vi "Test DISCONNECT packet.vi"(8 "error in":errorcluster) -> (0 "error out":errorcluster)   [LabVIEW 2013]
uses:
  source/Control Packets/DISCONNECT/DISCONNECT.lvclass
  source/Control Packets/ControlPacket/ControlPacket.lvclass/ControlPacket.ctl
  source/Control Packets/ControlPacket/ControlPacket.lvclass
  <vilib>/addons/_JKI Toolkits/Caraya/classes/Test/Test.lvclass
  <vilib>/addons/_JKI Toolkits/Caraya/classes/Assert/Assert.lvclass
panel:
  out "Packet ID":u16 format="%04x"
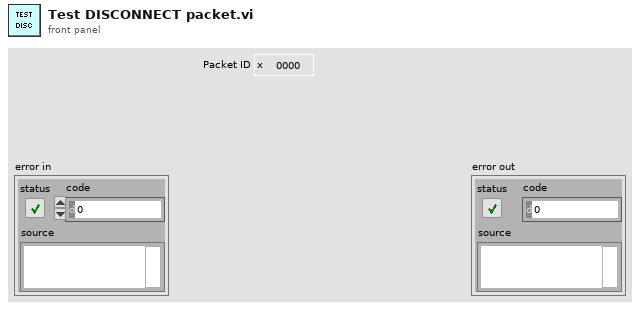
[diagram p1: front panel]
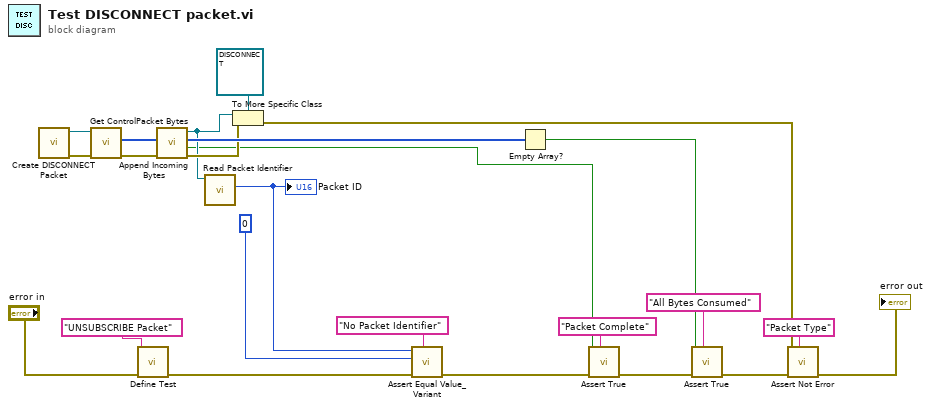
[diagram p0: block diagram]
diagram:
  n1 = call "Create DISCONNECT Packet.vi"() -> ("error out"=w18:errorcluster, "DISCONNECT"=w19:refnum<class "DISCONNECT.lvclass">)  [unwired: 10 in]
  n2 = call "Get ControlPacket Bytes.vi"("error in (no error)"=w18, "ControlPacket"=w19) -> ("error out"=w22:errorcluster, "Bytes Stream"=w24:u8[])  [unwired: 6 in, 2 out]
  n3 = call <vilib>:"Define Test.vi"("error in (no error)"="error in", "Label (VI Title)"="UNSUBSCRIBE Packet") -> ("error out"=w11:errorcluster)  [unwired: 9 in]
  n4 = call "Append Incoming Bytes.vi"("error in (no error)"=w22, "Incoming Packets"=w24) -> ("error out"=w21:errorcluster, "Complete Packet"=w4:bool, "Remaining Packets"=w23:u8[], "ControlPacket"=w20:refnum<class "ControlPacket.lvclass">)  [unwired: 6 in]
  n5 = call "Read Packet Identifier.vi"("ControlPacket in"=w20) -> ("Packet Identifier"=w2:u16)  [unwired: 9 in, 1 out]
  "Packet ID" <- w2
  n6 = To More Specific Class(target class=refnum<class "DISCONNECT.lvclass"> refnum ("MQTT_Control_Packets.lvlib:DISCONNECT.lvclass"), reference=w20, error in=w21) -> (error out=w6:errorcluster)  [unwired: 1 out]
  n7 = call <vilib>:"Assert Equal Value_Variant.vi"("Label"="No Packet Identifier" ("Label (VI Title)"), "error in (no error)"=w11, "Y"=u16 0 ("y"), "X"=w2) -> ("error out"=w3:errorcluster)  [unwired: 7 in]
  n8 = Empty Array?(array=w23) -> (empty?=w5:bool)
  n9 = call <vilib>:"Assert True.vi"("Label"="Packet Complete" ("Label (VI Title)"), "error in (no error)"=w3, "True?"=w4) -> ("error out"=w12:errorcluster)  [unwired: 8 in]
  n10 = call <vilib>:"Assert True.vi"("Label"="All Bytes Consumed" ("Label (VI Title)"), "error in (no error)"=w12, "True?"=w5) -> ("error out"=w9:errorcluster)  [unwired: 8 in]
  n11 = call <vilib>:"Assert Not Error.vi"("Label"="Packet Type" ("Label (VI Title)"), "error in (no error)"=w9, "Not Error?"=w6) -> ("error out"=→"error out":errorcluster)  [unwired: 8 in]
